vi "Mapping Simulated Spectrum v10.6.4.vi"() -> (0 "Simulated Spectrum":cluster{i32[], dbl[]}[](array[cluster]))   [LabVIEW 2010]
panel:
  out "Spectrum":cluster{i32[], dbl[]}[](graph)
  out "Y (1D)":dbl[](array[numeric])
  out "X (1D)":i32[](array[numeric])
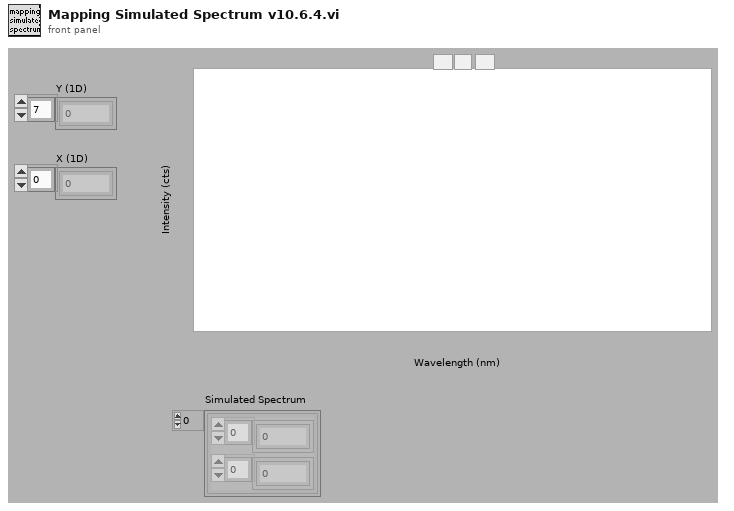
[diagram p1: front panel]
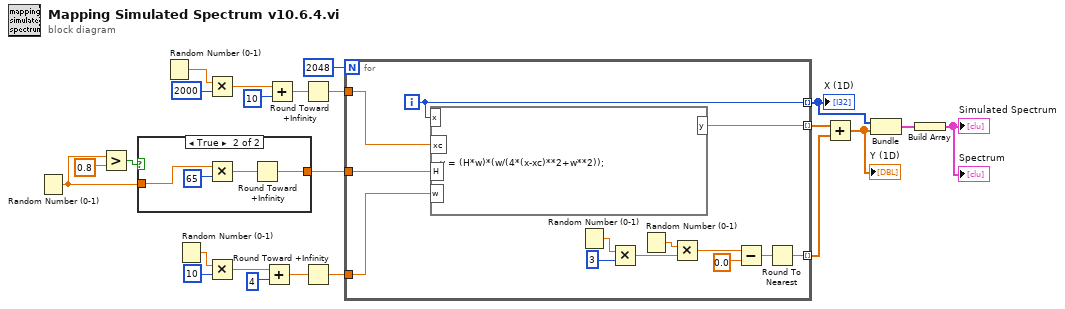
[diagram p0: block diagram]
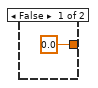
[diagram p2: hidden frame]
diagram:
  n1 = Random Number (0-1)() -> (number: 0 to 1=w5:dbl)
  n2 = Greater?(x=w5, y=0.8) -> (0:w6:bool)
  n3 = case shown="True" w6 {
    tunnel: w5 -> [_ w26]
    tunnel: [0.0 w25] -> w4
    frame False {
    }
    frame True {
      n4 = Multiply(x=w26, y=65) -> (x*y=w28:dbl)
      n5 = Round Toward +Infinity(x=w28) -> (ceil(x): smallest int >= x=w25:dbl)
    }
  }
  n6 = Random Number (0-1)() -> (number: 0 to 1=w21:dbl)
  n7 = Random Number (0-1)() -> (number: 0 to 1=w18:dbl)
  n8 = Multiply(x=w21, y=2000 ("Dimension")) -> (x*y=w11:dbl)
  n9 = Multiply(x=w18, y=10) -> (x*y=w16:dbl)
  n10 = Add(x=w16, y=4) -> (x+y=w15:dbl)
  n11 = Add(x=w11, y=10 ("Dimension")) -> (x+y=w9:dbl)
  n12 = Round Toward +Infinity(x=w9) -> (ceil(x): smallest int >= x=w8:dbl)
  n13 = Round Toward +Infinity(x=w15) -> (ceil(x): smallest int >= x=w13:dbl)
  n14 = for {
    N: 2048 ("Dimension") -> [_]
    tunnel: [w38] -> w22 mode=indexing
    tunnel: w13 -> [w41]
    tunnel: w4 -> [w40]
    tunnel: w8 -> [w39]
    tunnel: [w37] -> w3 mode=indexing
    tunnel: [w33] -> w1 mode=indexing
    i -> [w38]
    n15 = formula code="y = (H*w)*(w/(4*(x-xc)**2+w**2));"("x"=w38, "H"=w40, "w"=w41, "xc"=w39) -> ("y"=w37:dbl)
    n16 = Random Number (0-1)() -> (number: 0 to 1=w36:dbl)
    n17 = Multiply(x=w36, y=3 ("Dimension")) -> (x*y=w31:dbl)
    n18 = Random Number (0-1)() -> (number: 0 to 1=w32:dbl)
    n19 = Multiply(x=w32, y=w31) -> (x*y=w30:dbl)
    n20 = Subtract(x=w30, y=0.0) -> (x-y=w35:dbl)
    n21 = Round To Nearest(number=w35) -> (nearest integer value=w33:dbl)
  }
  "X (1D)" <- w22
  n22 = Add(x=w3, y=w1) -> (x+y=w2:dbl[])
  "Y (1D)" <- w2
  n23 = Bundle(w22, w2) -> (w23:cluster{i32[], dbl[]})  [unwired: 1 in]
  n24 = Build Array(w23) -> (→"Simulated Spectrum" →"Spectrum":cluster{i32[], dbl[]}[])
